vi "GLIMPSE Sequence Player.vi"() -> (8 "Sequence Range":cluster{i32, i32})   [LabVIEW 2016]
doc: "Allows the user to view and analyze a sequence of video stored as a temporary file on the disk. Also includes tools for setting areas of interest, manual tracking, automatic tracking by image fitting, etc."
uses:
  Header file data.ctl
  Seq file v 1/Offset table.ctl
  Seq file v 1/Offset.ctl
  Seq file v 1/file number.ctl
  Header2 file data.ctl
  <vilib>/vision/Image Controls.llb/IMAQ Image.ctl
  GLIMPSE Globals.vi
  <vilib>/Utility/file.llb/Write To Spreadsheet File (I64).vi
  AOI/AOI List Globals.vi
  <vilib>/Utility/NIReport.llb/NI_ReportGenerationCore.lvlib
panel:
  out "Header2 data":T1
  in  "Exit":bool
  out "Acquisition refnum array":refnum<file>[](array[refnum])
  out "file path":path
  out "Header data":T2 {"Pixel depth" items=["8 bits", "16 bits", "Float", "Complex", "RGB", "HSL"]; "time of 1st frame, \nsec since 1/1/04" format="%.2f"}
  in  "Change File":bool
  in  "Tab Control":T6(tab)
  in  "Overlay?":bool=TRUE caption="Loop?"
  in  "Frames to Step":u32=1 min=1 step=1
  in  "# Display\nWindows":i32=1 min=0 max=8 step=1
  in  "Delay between frames (msec)":i32=33 min=0 max=2147483600 step=100
  in  "Stop!":bool
  out "Time after 1st\nFrame (ms)":u32
  out "Mode":T7(ring)
  out "Time\nStamp":u32
  in  "Step Backward":bool
  in  "Step Forward":bool
  in  "Play Backward":bool
  in  "Play Forward":bool
  in  "Go to End":bool
  in  "Go to Begin":bool
  in  "Toggle beg/end":bool
  in  "Set end":bool
  in  "Set begin":bool
  in  "Loop?":bool=TRUE
  in  "Range Enabled":bool=TRUE caption="Restrict playback to range"
  in  "Frame Number":cluster{u32, u32}(slide)={10, 1} scale=1.0..3558.0
  in  "Current Frame Number":u32(slide) max=3558 scale=1.0..3558.0
  out "Rev bkd":bool
  out "Fwd bkd":bool
  out "Stop bkgd":bool
  out "Filter":u16
  out "Field":u16
  out "Lasers":bool[](array[boolean])
  out "Flow":dbl
  out "Temp":dbl
  in  "Total FOVs":i16=4
  in  "Display FOV number":i16(slide)=1 min=1 scale=1.0..4.0
  in  "FOV Mode":T8(ring)=enum."Display all frames"
  in  "Printer":u16(ring) items=["zippy", "Send To OneNote 2010", "prism", "Microsoft XPS Document Writer", "Fax"]
  in  "Track by Curve Fitting to AOIs":bool
  in  "Print Image":bool
  in  "Save Portion of Current Frame":bool
  in  "Save Sequence":bool
  in  "Set/Modify AOIs (F8)":bool
  in  "Clear All":bool
  in  "Erase Last Row":bool
  out "Tracking Output File":path
  out "Number of Points":i16
  in  "Table":string[][](table)
  out "Pixel depth":u32(ring) items=["8 bits", "16 bits", "Float", "Complex", "RGB", "HSL"]
  out "Number of Frames":u32
  out "Frame width":i32
  out "Frame height":i32
  out "Camera":string
  out "Microscope":string
  out "Microscope software version":string
  out "Filter names":string[](array[string])
  out "Laser names":string[](array[string])
  # "These parameters are not for interactive use:"
  # "1"
  # "1"
  # "(F1)"
  # "(F2)"
  # "(F3)"
  # "(F4)"
  # "(F12)"
  # "Begin"
  # "Set"
  # "End"
  # "To add an (X, Y, T) point to table, click on image #1 with the point tool (\"+\")."
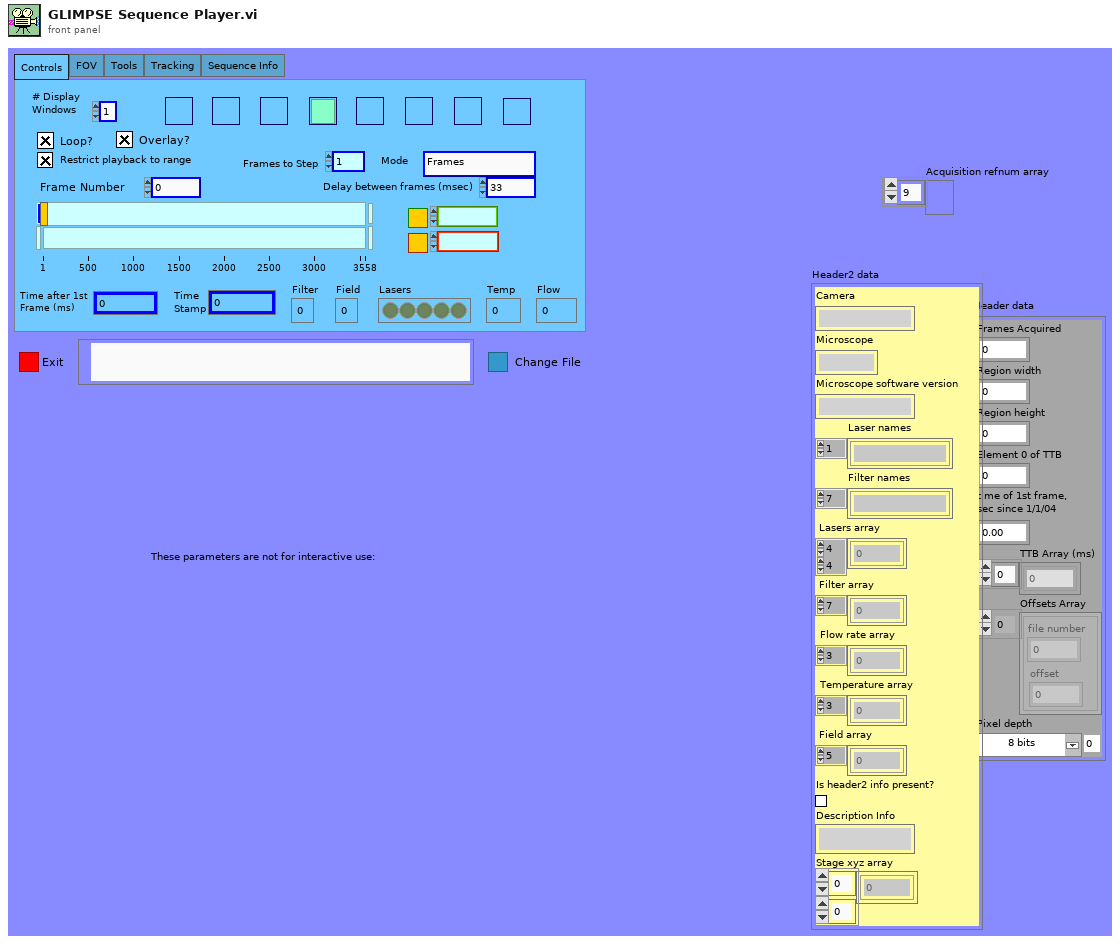
[diagram p1: front panel]
types:
  T1 = typedef "Header2 file data.ctl" = cluster{"Camera":string, "Microscope":string, "Microscope software version":string, "Laser names":string[], "Filter names":string[], "Lasers array":u16[][], "Filter array":u16[], "Flow rate array":dbl[], "Temperature array":dbl[], "Field array":u16[], "Is header2 info present?":bool, "Description Info":string, "Stage xyz array":dbl[][]}
  T2 = typedef "Header file data.ctl" = cluster{"Frames Acquired":u32, "Region width":i32, "Region height":i32, "Element 0 of TTB":u32, "time of 1st frame, \nsec since 1/1/04":dbl, "TTB Array (ms)":u32[], "Offsets Array":T3, "Pixel depth":u32}
  T3 = typedef "Offset table.ctl" = cluster{"offset":T4, "file number":T5}[]
  T4 = typedef "Offset.ctl" = i32
  T5 = typedef "file number.ctl" = u8
  T6 = enum32{"Controls", "FOV", "Tools", "Tracking", "Sequence Info"}
  T7 = enum16{"Frames", "Fields, Odd 1st", "Fields, Even 1st", "Fields, Averaged"}
  T8 = enum16{"Display one field of view", "Display all frames"}
  T9 = typedef "IMAQ Image.ctl" = refnum<image>
  T10 = enum32{"No Selection", "Point", "Line", "Rectangle", "Oval", "Polygon", "Free", "Unused1", "Zoom", "Unused2", "Broken Line", "Free Hand Line"}
  T11 = enum32{"No  event", "Click event", "Draw event", "Move event", "Size event", "Scroll event", "Activate event", "Close event", "Reserved"}[]
  T12 = cluster{"# of Frames Out (Log)":u32, "Current Frame Number":u32}
  T13 = cluster{"Left":i32, "Top":i32, "Right":i32, "Bottom":i32}
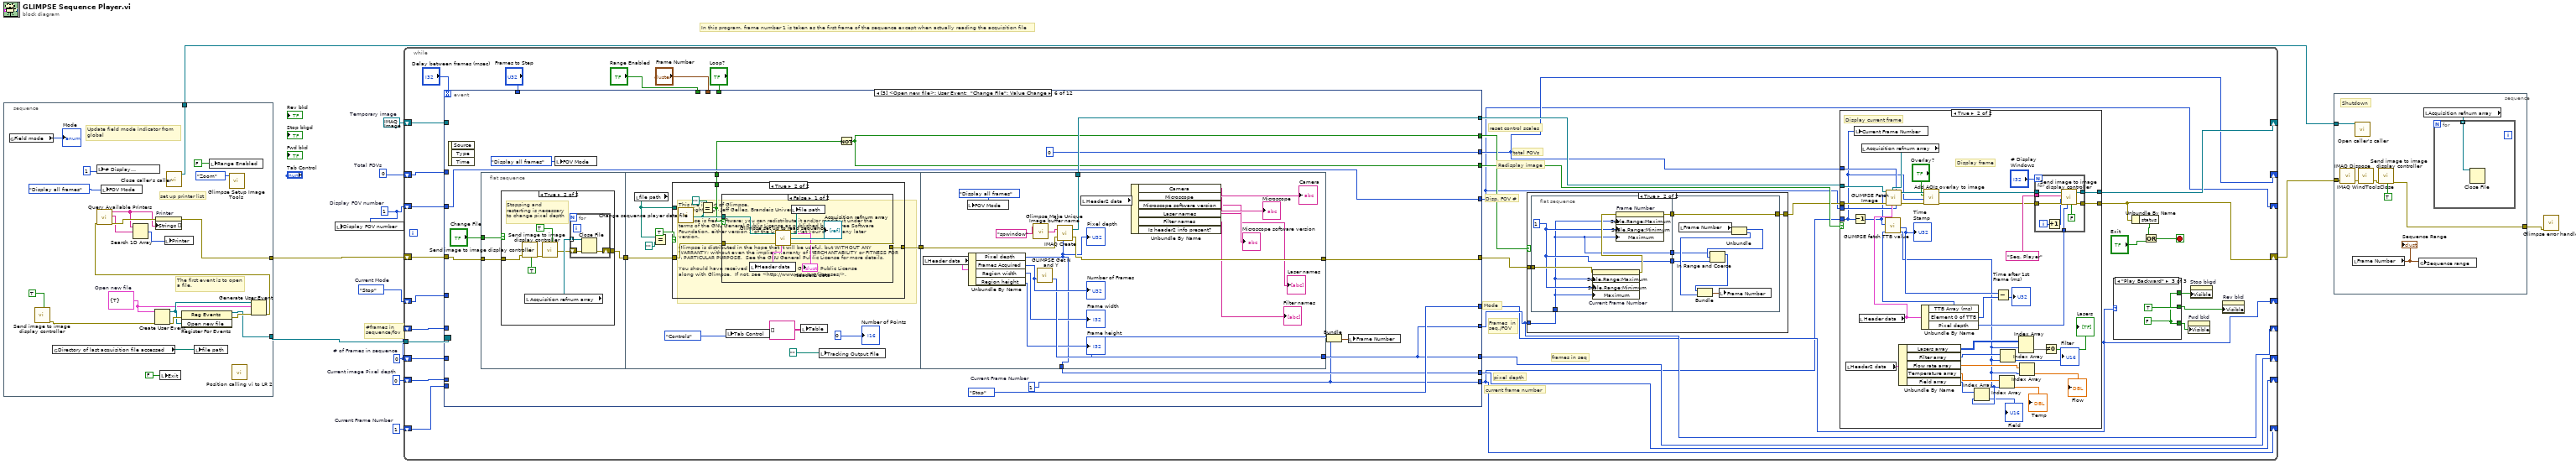
[diagram p0: block diagram]
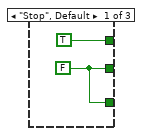
[diagram p2: hidden frame]
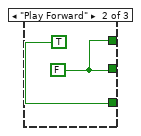
[diagram p3: hidden frame]
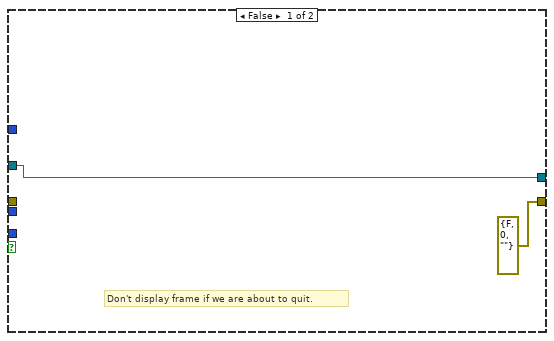
[diagram p4: hidden frame]
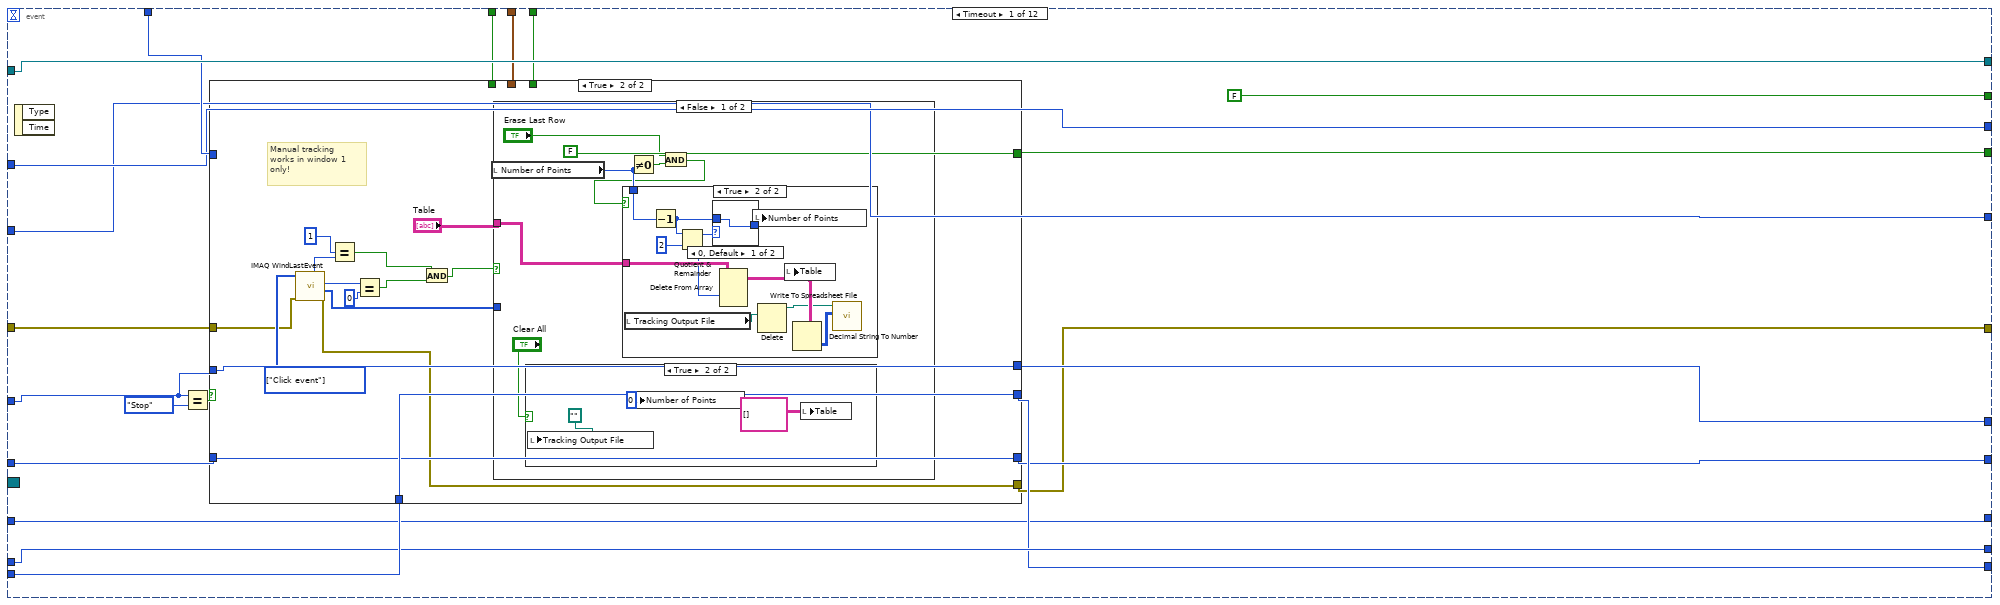
[diagram p6: hidden frame]
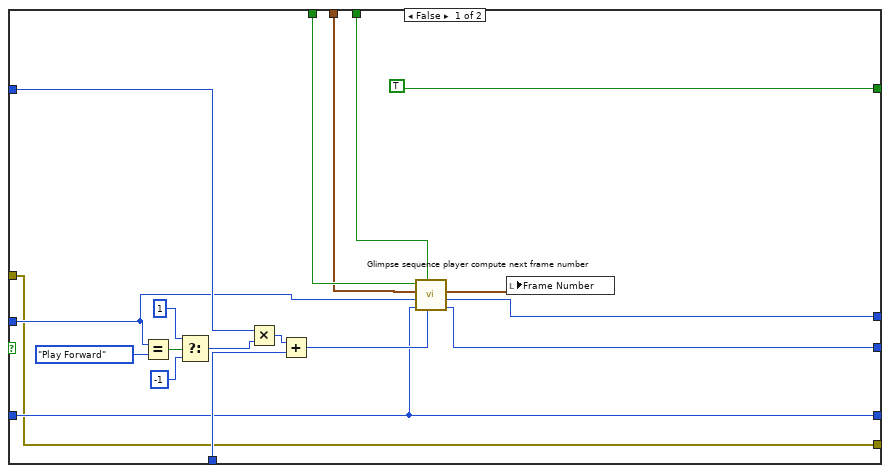
[diagram p7: hidden frame]
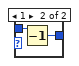
[diagram p10: hidden frame]
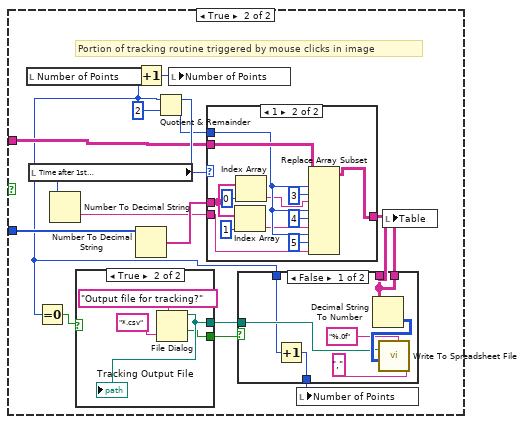
[diagram p11: hidden frame]
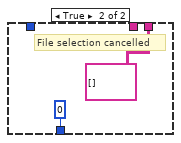
[diagram p12: hidden frame]
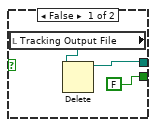
[diagram p13: hidden frame]
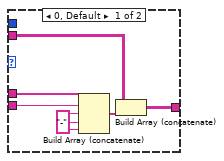
[diagram p14: hidden frame]
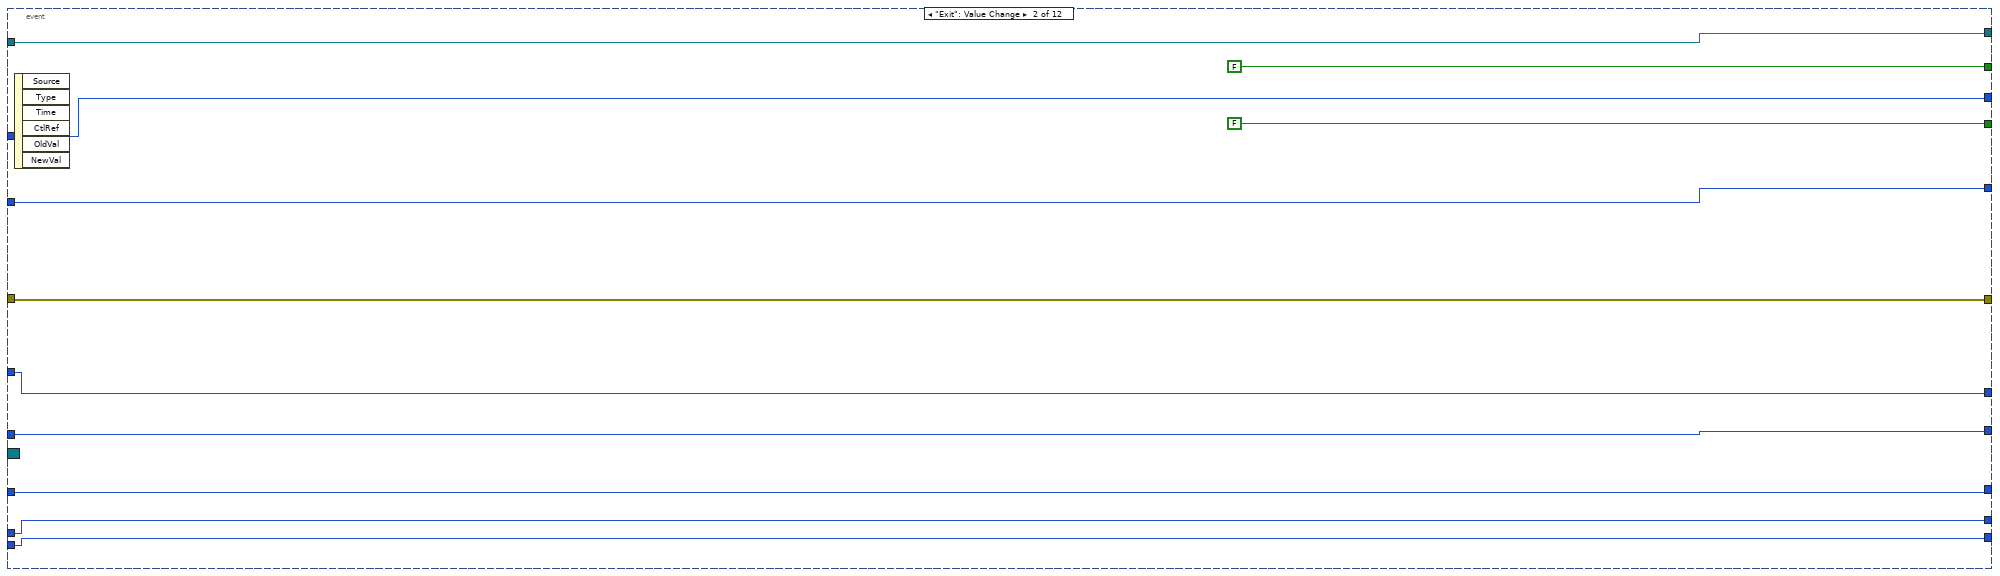
[diagram p15: hidden frame]
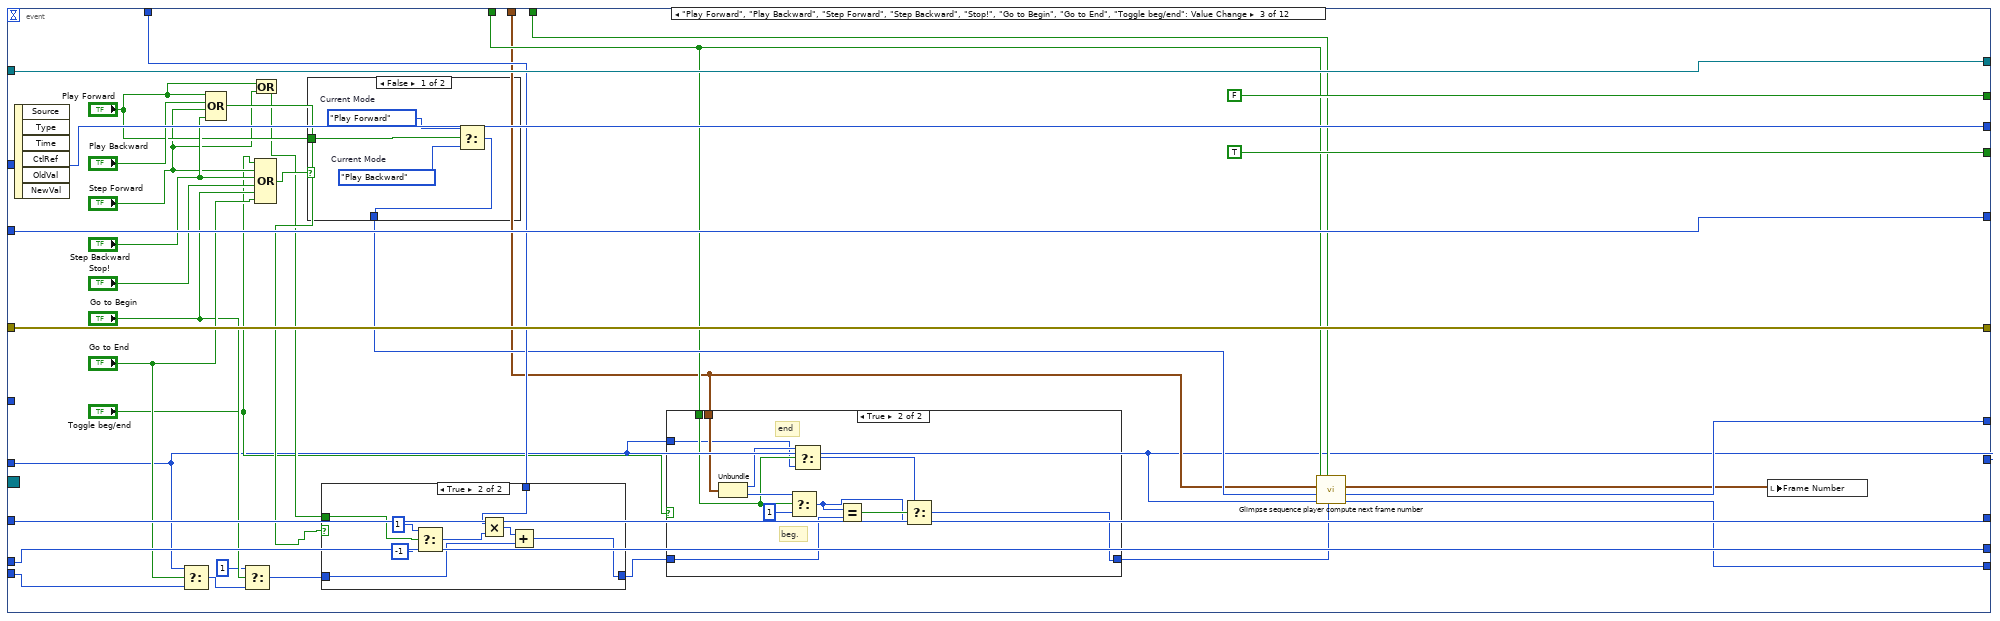
[diagram p16: hidden frame]
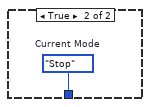
[diagram p19: hidden frame]
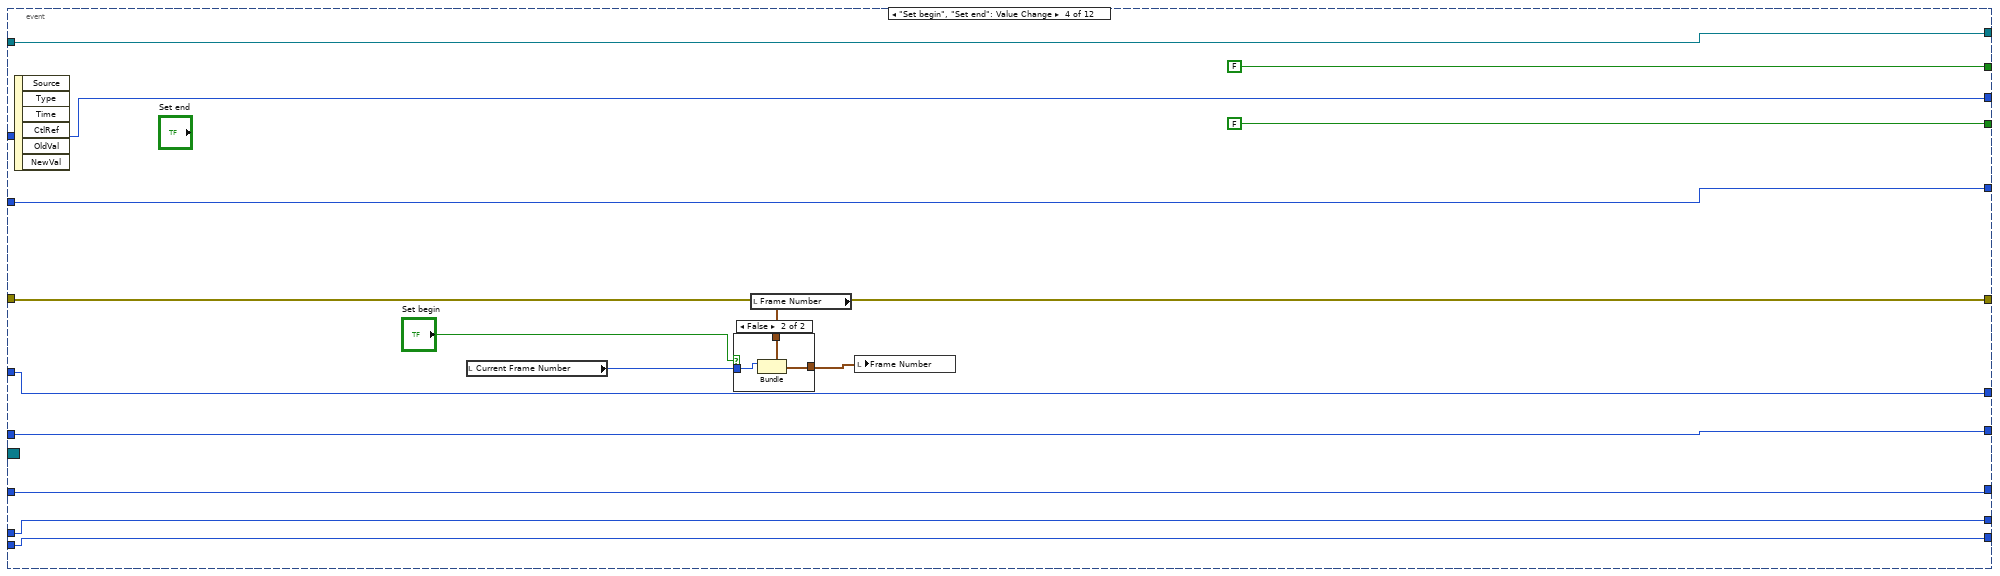
[diagram p20: hidden frame]
diagram:
  w3 = u32 0  # # of Frames in sequence
  w6 = T9 refnum  # Temporary image
  w4 = i16 1  # Display FOV number
  w7 = i16 0  # Total FOVs
  w8 = u32 0  # Current image Pixel depth
  w11 = u32 1  # Current Frame Number
  w5 = enum16{"Stop", "Play Forward", "Play Backward"}."Stop"  # Current Mode
  # "This file is part of Glimpse. \nCopyright 2014 Jeff Gelles, Brandeis University.    \n\nGlimpse is free software: you can redistribute it and/or modify it under the \nterms of the GNU General Public License as published by the Free Software \nFoundation, either version 3 of the License, or (at your option) any later \nversion.\n\nGlimpse is distributed in the hope that it will be useful, but WITHOUT ANY \nWARRANTY; without even the implied warranty of MERCHANTABILITY or FITNESS FOR \nA PARTICULAR PURPOSE.  See the GNU General Public License for more details.\n\nYou should have received a copy of the GNU General Public License\nalong with Glimpse.  If not, see <http://www.gnu.org/licenses/>."
  # "#frames in\nsequence/fov"
  # "In this program, frame number 1 is taken as the first frame of the sequence except when actually reading the acquisition file"
  n1 = stacked-sequence {
    tunnel: [w32] -> w12
    tunnel: [w21] -> w10
    tunnel: [w17] -> w9
    frame #0 {
      w14 = cluster{"dummy":bool} {"dummy"=TRUE}  # Open new file
      # "Update field mode indicator from\nglobal"
      # "The first event is to open\na file."
      # "set up printer list"
      n2 = global read "GLIMPSE Globals.vi" "Field mode"() -> (→"Mode":T7)
      n3 = call "Send image to image display controller.vi"("Start display controller?"=TRUE ("Quit display controller?")) -> ("error out"=w18:errorcluster)  [unwired: 6 in, 3 out]
      n4 = global read "GLIMPSE Globals.vi" "Directory of last acquisition file accessed"() -> (w25:path)
      n5 = local write "# Display\nWindows"(1 ("# Display\nWindows")) -> ()
      n6 = local write "FOV Mode"(T8."Display all frames" ("FOV Mode")) -> ()
      n7 = Create User Event(user event datatype=w14, error in=w18) -> (user event=w22:refnum<user-event>, error out=w24:errorcluster)
      n8 = local write "Exit"(FALSE ("Exit")) -> ()
      n9 = call "Close caller's caller.vi"() -> ("vi reference"=w32:refnum<vi>)  [unwired: 1 in, 7 out]
      n10 = register-events(error in=w24, w22) -> (reference out=w21:refnum<event-registration>, error out=w23:errorcluster)  [unwired: 1 in]
      n11 = local write "file path"(w25) -> ()
      n12 = local write "Range Enabled"(FALSE ("Exit")) -> ()
      n13 = call "Glimpse Setup Image Tools"("Default Tool"=T10."Zoom") -> ()  [unwired: 1 in, 3 out]
      n14 = call "Position calling vi to LR 2.vi"() -> ()  [unwired: 2 in, 4 out]
      n15 = Generate User Event(user event=w22, event data cluster=w14, error in=w23) -> (error out=w20:errorcluster)  [unwired: 1 in, 1 out]
      n16 = call <vilib>:"Query Available Printers.vi"("error in (no error)"=w20) -> ("error out"=w30:errorcluster, "default printer"=w29:string, "system configured printers"=w28:string[])  [unwired: 8 out]
      n17 = Search 1D Array(1D array=w28, element=w29) -> (index of element=w27:i32)  [unwired: 1 out]
      n18 = property on="Printer" class="Ring (strict)"(error in=w30, "Strings []"=w28) -> (error out=w17:errorcluster)  [unwired: 1 in, 1 out]
      n19 = local write "Printer"(w27) -> ()
    }
  }
  n20 = local write "Display FOV number"(w4) -> ()
  n21 = while {
    shift-right: [w34] -> _
    shift-left: w11 -> [w66]
    tunnel: w10 -> [w68]
    shift-right: [w43] -> w2
    shift-left: w9 -> [w67]
    shift-right: [w56] -> _
    shift-left: w6 -> [w61]
    shift-right: [w65] -> _
    shift-left: w8 -> [w64]
    shift-right: [w47] -> _
    shift-left: w7 -> [w63]
    shift-right: [w46] -> _
    shift-left: w4 -> [w62]
    shift-right: [w38] -> _
    shift-left: w5 -> [w60]
    shift-right: [w55] -> _
    shift-left: w3 -> [w59]
    shift-right: [w39] -> _
    shift-left: w3 -> [w45]
    stop <- w44 stop-if-true
    (unwired) cluster{string, u32}[] [] ("Images")
    # "pixel depth"
    # "frames in seq"
    # "Frames  in\nseq./FOV"
    # "Mode"
    # "Disp. FOV #"
    # "total FOVs"
    # "current frame number"
    # "Redisplay image"
    # "reset control scales"
    n22 = event shown="[5] <Open new file>: User Event;  \"Change File\": Value Change" {
      selector: w68 -> [_ _ _ _ _ _ _ _ _ _ _ _]
      dyn-events: _ -> [_ _ _ _ _ _ _ _ _ _ _ _]
      timeout: "Delay between frames (msec)" -> [_ _ _ _ _ _ _ _ _ _ _ _]
      tunnel: w67 -> [w142 w273 w310 w348 w367 w399 w505 w528 w552 w581 w595 w623]
      tunnel: [w159 w280 w314 w355 w373 w396 w467 w530 w551 w585 w596 w624] -> w57
      tunnel: [w141 w273 w310 w348 w367 w395 w474 w528 w539 w581 w594 w623] -> w49
      tunnel: [FALSE ("Reset control scales?") FALSE ("Reset control scales?") FALSE ("Reset control scales?") FALSE ("Reset control scales?") FALSE ("Reset control scales?") w384 w472 w532 w554 w587 TRUE ("Reset control scales?") w628] -> w58
      tunnel: w66 -> [w154 w279 w303 w354 w372 _ w464 w534 w549 w584 w602 _]
      tunnel: [w151 w279 w291 w354 w372 w387 w464 w534 w549 w584 w599 "Current Frame Number"] -> w34
      tunnel: [w152 w278 w313 w353 w371 w392 w475 w533 w548 w583 w600 w626] -> w65
      tunnel: w64 -> [w152 w278 w313 w353 w371 _ w475 w533 w548 w583 w600 w626]
      tunnel: w63 -> [w153 w270 w307 w345 w364 _ w470 w529 w544 w580 _ w619]
      tunnel: w62 -> [w144 w274 w311 w349 w368 w390 w469 w527 w541 w578 _ w620]
      tunnel: w61 -> [w159 w280 w314 w355 w373 _ w468 w530 w551 w585 w596 w624]
      tunnel: w60 -> [w156 w275 _ w350 _ _ _ _ w550 w579 w593 w622]
      tunnel: [w146 w275 w289 w350 w362 enum16{"Stop", "Play Forward", "Play Backward"}."Stop" ("Current Mode") enum16{"Stop", "Play Forward", "Play Backward"}."Stop" ("Current Mode") enum16{"Stop", "Play Forward", "Play Backward"}."Stop" ("Current Mode") w550 w579 w593 w622] -> w38
      tunnel: [w145 w277 w312 w352 w370 w388 w465 w525 w547 w582 w598 w625] -> w55
      tunnel: w59 -> [w145 w277 w312 w352 w370 _ w465 w525 w547 w582 w598 w625]
      tunnel: [w153 w270 w307 w345 w364 i16 0 ("Total FOVs") w470 w529 w544 w580 w606 w619] -> w47
      tunnel: [w144 w274 w311 w349 w368 w390 w469 w527 w541 w578 w605 w620] -> w46
      tunnel: [w143 w276 w281 w351 w369 w388 w466 w526 w546 w577 w603 w621] -> w39
      tunnel: [w157 FALSE ("Redisplay image") TRUE ("Redisplay image") FALSE ("Redisplay image") FALSE ("Redisplay image") w384 w471 w531 w553 w586 TRUE ("Redisplay image") w627] -> w50
      tunnel: w45 -> [w150 w276 w281 w351 w369 _ w466 w526 w546 w577 _ w621]
      tunnel: "Frames to Step" -> [w155 _ w295 _ _ _ _ _ _ _ _ _]
      tunnel: "Loop?" -> [w149 _ w288 _ _ _ _ _ _ _ _ _]
      tunnel: "Range Enabled" -> [w148 _ w283 _ _ _ _ _ _ _ _ _]
      tunnel: "Frame Number" -> [w147 _ w282 _ w363 _ _ _ _ _ _ _]
      event Timeout {
        n23 = event-data() -> ()  [unwired: 3 out]
        n24 = Equal?(x=w156, y=enum16{"Stop", "Play Forward", "Play Backward"}."Stop") -> (x = y?=w161:bool)
        n25 = case shown="True" w161 {
          tunnel: [TRUE ("Reset control scales?") FALSE ("Reset control scales?")] -> w157
          tunnel: w156 -> [w167 w194]
          tunnel: w155 -> [w177 _]
          tunnel: w154 -> [w172 w195]
          tunnel: [w165 w195] -> w151
          tunnel: w150 -> [w163 w193]
          tunnel: w149 -> [w170 _]
          tunnel: w148 -> [w169 _]
          tunnel: w147 -> [w168 _]
          tunnel: [w164 w194] -> w146
          tunnel: [w163 w193] -> w143
          tunnel: w142 -> [w162 w182]
          tunnel: [w162 w181] -> w141
          frame False {
            n26 = Equal?(x=w167, y=enum16{"Stop", "Play Forward", "Play Backward"}."Play Forward") -> (x = y?=w178:bool)
            n27 = Select(t=1, s=w178, f=-1) -> (s? t:f=w176:i32)
            n28 = Multiply(x=w177, y=w176) -> (x*y=w173:u32)
            n29 = Add(x=w173, y=w172) -> (x+y=w166:u32)
            n30 = call "Glimpse sequence player compute next frame number.vi"("Current Frame Number"=w166, "Loop?"=w170, "# of Frames in sequence/FOV"=w163, "Current Mode"=w167, "Range In"=w168, "Range Enabled"=w169) -> ("Current Frame Number Out"=w165:u32, "Current Mode Out"=w164:enum16{"Stop", "Play Forward", "Play Backward"}, "Range Out"=w171:cluster{"Max":u32, "Min":u32})  [unwired: 1 out]
            n31 = local write "Frame Number"(w171) -> ()
          }
          frame True {
            w191 = T11 [enum."Click event"] items=["No  event", "Click event", "Draw event", "Move event", "Size event", "Scroll event", "Activate event", "Close event", "Reserved"] ("Events list (all)")
            # "Manual tracking \nworks in window 1\nonly!"
            n32 = call "IMAQ WindLastEvent"("error in (no error)"=w182, "Events list (all)"=w191) -> ("error out"=w181:errorcluster, "Coordinates"=w185:i32[], "Tool"=w190:i32, "Window Number (0...15)"=w192:i32)  [unwired: 6 out]
            n33 = Equal?(x=1 ("Window Number (0...15)"), y=w192) -> (x = y?=w187:bool)
            n34 = Equal?(x=w190, y=0) -> (x = y?=w188:bool)
            n35 = And(x=w187, y=w188) -> (x .and. y?=w186:bool)
            n36 = case shown="False" w186 {
              tunnel: w185 -> [_ w231]
              tunnel: "Table" -> [w201 w225]
              frame False {
                n37 = local read "Number of Points"() -> (w200:i16)
                n38 = case shown="True" "Clear All" {
                  frame False {
                  }
                  frame True {
                    n39 = local write "Tracking Output File"(path "") -> ()
                    n40 = local write "Number of Points"(i16 0 ("Number of Points")) -> ()
                    n41 = local write "Table"(string[][] []) -> ()
                  }
                }
                n42 = Not Equal To 0?(x=w200) -> (x != 0?=w199:bool)
                n43 = And(x="Erase Last Row", y=w199) -> (x .and. y?=w198:bool)
                n44 = case shown="True" w198 {
                  tunnel: w201 -> [_ w212]
                  tunnel: w200 -> [_ w207]
                  frame False {
                  }
                  frame True {
                    n45 = local read "Tracking Output File"() -> (w206:path)
                    n46 = Decrement(x=w207) -> (x-1=w215:i16)
                    n47 = Quotient & Remainder(x=w215, y=i16 2) -> (x-y*floor(x/y)=w213:i16, floor(x/y)=w211:i16)
                    n48 = case shown="0, Default" w213 {
                      tunnel: w215 -> [w217 w219]
                      tunnel: [w217 w218] -> w214
                      frame 0, Default {
                      }
                      frame 1 {
                        n49 = Decrement(x=w219) -> (x-1=w218:i16)
                      }
                    }
                    n50 = Delete From Array(array=w212, index (row)=w211) -> (array with subset deleted=w210:string[][])  [unwired: 2 in, 1 out]
                    n51 = local write "Number of Points"(w214) -> ()
                    n52 = Delete(path (use dialog)=w206) -> (deleted path=w209:path)  [unwired: 1 in, 5 out]
                    n53 = local write "Table"(w210) -> ()
                    n54 = Decimal String To Number(string=w210) -> (number=w208:i32[][])  [unwired: 3 out]
                    n55 = call-poly <vilib>:"Write To Spreadsheet File.vi"("2D data"=w208, "file path (dialog if empty)"=w209) -> ()  [unwired: 4 in, 3 out]
                  }
                }
              }
              frame True {
                # "Portion of tracking routine triggered by mouse clicks in image"
                n56 = local read "Number of Points"() -> (w222:i16)
                n57 = local read "Time after 1st\nFrame (ms)"() -> (w232:u32)
                n58 = Equal To 0?(x=w222) -> (x = 0?=w227:bool)
                n59 = Number To Decimal String(number=w232) -> (decimal integer string=w229:string)  [unwired: 1 out]
                n60 = case shown="True" w227 {
                  tunnel: [w246 w249] -> w223
                  tunnel: [FALSE ("cancelled") w248] -> w224
                  frame False {
                    n61 = local read "Tracking Output File"() -> (w247:path)
                    n62 = Delete(path (use dialog)=w247) -> (deleted path=w246:path)  [unwired: 1 in, 5 out]
                  }
                  frame True {
                    n63 = File Dialog(6:"*.csv" ("pattern"), 7:"Output file for tracking?" ("prompt")) -> (1:w248:bool, 3:w249:path)  [unwired: 1 in, 6 out]
                    "Tracking Output File" <- w249
                  }
                }
                n64 = Increment(x=w222) -> (x+1=w234:i16)
                n65 = Number To Decimal String(number=w231) -> (decimal integer string=w230:string[])  [unwired: 1 in]
                n66 = Quotient & Remainder(x=w222, y=i16 2) -> (x-y*floor(x/y)=w233:i16, floor(x/y)=w228:i16)
                n67 = local write "Number of Points"(w234) -> ()
                n68 = case shown="1" w233 {
                  tunnel: w225 -> [w257 w269]
                  tunnel: [w254 w268] -> w226
                  tunnel: w230 -> [w253 w262]
                  tunnel: w229 -> [w252 w263]
                  tunnel: w228 -> [_ w264]
                  frame 0, Default {
                    w255 = "-"
                    n69 = Build Array (concatenate)(w253, w252, w255, w255, w255) -> (w256:string[])
                    n70 = Build Array (concatenate)(w257, w256) -> (w254:string[][])
                  }
                  frame 1 {
                    n71 = Index Array(array=w262, index=1 ("Index")) -> (element=w258:string)
                    n72 = Index Array(array=w262, index=0 ("Index")) -> (element=w259:string)
                    n73 = Replace Array Subset(array=w269, new element #1=w259, index (row) #1=w264, index (col) #1=3 ("Disabled Index (col)"), new element #2=w258, index (row) #2=w264, index (col) #2=4 ("Index (col)"), new element #3=w263, index (row) #3=w264, index (col) #3=5 ("Index (col)")) -> (w268:string[][])
                  }
                }
                n74 = case shown="False" w224 {
                  tunnel: w226 -> [w238 _]
                  tunnel: w223 -> [w241 _]
                  tunnel: w222 -> [w240 _]
                  tunnel: [w239 i16 0] -> w221
                  tunnel: [w238 string[][] []] -> w220
                  frame False {
                    n75 = Increment(x=w240) -> (x+1=w239:i16)
                    n76 = Decimal String To Number(string=w238) -> (number=w242:i32[][])  [unwired: 3 out]
                    n77 = call-poly <vilib>:"Write To Spreadsheet File.vi"("delimiter (\\t)"="," ("delimiter (Tab)"), "format (%d)"="%.0f" ("format (%.3f)"), "2D data"=w242, "file path (dialog if empty)"=w241) -> ()  [unwired: 3 in, 2 out]
                  }
                  frame True {
                    # "File selection cancelled"
                  }
                }
                n78 = local write "Number of Points"(w221) -> ()
                n79 = local write "Table"(w220) -> ()
              }
            }
          }
        }
      }
      event "Exit": Value Change {
        n80 = event-data() -> ()  [unwired: 7 out]
      }
      event "Play Forward", "Play Backward", "Step Forward", "Step Backward", "Stop!", "Go to Begin", "Go to End", "Toggle beg/end": Value Change {
        n81 = event-data() -> ()  [unwired: 7 out]
        n82 = Select(t=w281, s="Go to End", f=w303) -> (s? t:f=w301:u32)
        n83 = Compound Arithmetic op=OR("Play Forward", "Play Backward", "Step Forward", "Step Backward") -> (w297:bool)
        n84 = Select(t=u32 1, s="Go to Begin", f=w301) -> (s? t:f=w296:u32)
        n85 = Or(x="Play Forward", y="Step Forward") -> (x .or. y?=w292:bool)
        n86 = Compound Arithmetic op=OR("Toggle beg/end", "Step Forward", "Step Backward", "Stop!", "Go to Begin", "Go to End") -> (w305:bool)
        n87 = case shown="False" w305 {
          tunnel: [w336 w340] -> w290
          tunnel: "Play Forward" -> [w339 _]
          frame False {
            w337 = enum16{"Stop", "Play Forward", "Play Backward"}."Play Backward"  # Current Mode
            w338 = enum16{"Stop", "Play Forward", "Play Backward"}."Play Forward"  # Current Mode
            n88 = Select(t=w338, s=w339, f=w337) -> (s? t:f=w336:enum16{"Stop", "Play Forward", "Play Backward"})
          }
          frame True {
            w340 = enum16{"Stop", "Play Forward", "Play Backward"}."Stop"  # Current Mode
          }
        }
        n89 = case shown="True" w297 {
          tunnel: w296 -> [w327 w330]
          tunnel: [w327 w329] -> w285
          tunnel: w295 -> [_ w331]
          tunnel: w292 -> [_ w328]
          frame False {
          }
          frame True {
            n90 = Select(t=1, s=w328, f=-1) -> (s? t:f=w333:i32)
            n91 = Multiply(x=w331, y=w333) -> (x*y=w335:u32)
            n92 = Add(x=w335, y=w330) -> (x+y=w329:u32)
          }
        }
        n93 = case shown="True" "Toggle beg/end" {
          tunnel: w285 -> [w315 w325]
          tunnel: [w315 w316] -> w284
          tunnel: w283 -> [_ w320]
          tunnel: w282 -> [_ w323]
          tunnel: w281 -> [_ w318]
          frame False {
          }
          frame True {
            # "end"
            # "beg."
            n94 = Unbundle(w323) -> (w319:u32, w322:u32)
            n95 = Select(t=w322, s=w320, f=u32 1) -> (s? t:f=w321:u32)
            n96 = Select(t=w319, s=w320, f=w318) -> (s? t:f=w317:u32)
            n97 = Equal?(x=w321, y=w325) -> (x = y?=w324:bool)
            n98 = Select(t=w317, s=w324, f=w321) -> (s? t:f=w316:u32)
          }
        }
        n99 = call "Glimpse sequence player compute next frame number.vi"("Current Frame Number"=w284, "Loop?"=w288, "# of Frames in sequence/FOV"=w281, "Current Mode"=w290, "Range In"=w282, "Range Enabled"=w283) -> ("Current Frame Number Out"=w291:u32, "Current Mode Out"=w289:enum16{"Stop", "Play Forward", "Play Backward"}, "Range Out"=w287:cluster{"Max":u32, "Min":u32})  [unwired: 1 out]
        n100 = local write "Frame Number"(w287) -> ()
      }
      event "Set begin", "Set end": Value Change {
        n101 = event-data() -> ()  [unwired: 7 out]
        n102 = local read "Current Frame Number"() -> (w343:u32)
        n103 = local read "Frame Number"() -> (w342:cluster{u32, u32})
        n104 = case shown="False" "Set begin" {
          tunnel: [w358 w361] -> w344
          tunnel: w343 -> [w357 w359]
          tunnel: w342 -> [w356 w360]
          frame True {
            n105 = Bundle(cluster=w356, w357) -> (w358:cluster{u32, u32})  [unwired: 1 out]
          }
          frame False {
            n106 = Bundle(cluster=w360, w359) -> (w361:cluster{u32, u32})  [unwired: 1 out]
          }
        }
        n107 = local write "Frame Number"(w344) -> ()
      }
      event "Track by Curve Fitting to AOIs": Value Change {
        n108 = event-data() -> ()  [unwired: 7 out]
        n109 = flat-sequence {
          tunnel: [enum16{"Stop", "Play Forward", "Play Backward"}."Stop" ("Current Mode")] -> w362
          tunnel: w363 -> [w374]
          frame #0 {
            n110 = global read "GLIMPSE Globals.vi" "Current window Black/White Levels"() -> (w375:cluster{ext, ext})
            n111 = local read "Acquisition refnum array"() -> (w381:refnum<file>[])
            n112 = local read "Header data"() -> (w376:T2)
            n113 = Unbundle(w374) -> (w380:u32, w379:u32)
            n114 = Unbundle(w375) -> (w378:ext, w377:ext)
            n115 = call "fit aois.vi"("End frame"=w380, "White level"=w377, "Header Info"=w376, "Start frame"=w379, "Black level"=w378, "Acquisition refnum array"=w381) -> ()  [unwired: 5 out]
          }
          frame #1 {
            n116 = call "IMAQ WindToolsShow"() -> ("error out"=w383:errorcluster)  [unwired: 3 in, 3 out]
            n117 = call <vilib>:"Simple Error Handler.vi"("error in (no error)"=w383) -> ()  [unwired: 1 in, 8 out]
          }
        }
      }
      event User Event; "Change File": Value Change {
        w387 = u32 1  # Current Frame Number
        n118 = event-data() -> ()  [unwired: 4 out]
        n119 = flat-sequence {
          tunnel: w399 -> [w402]
          tunnel: [w401] -> w398
          tunnel: "Change File" -> [w400]
          tunnel: w398 -> [w421]
          tunnel: [w416] -> w397
          tunnel: [w414] -> w385
          tunnel: w397 -> [w460]
          tunnel: [w459] -> w396
          tunnel: [w458] -> w395
          tunnel: [w452] -> w392
          tunnel: [w456] -> w388
          frame #0 {
            n120 = case shown="True" w400 {
              tunnel: w402 -> [w403 w408]
              tunnel: [w403 w407] -> w401
              frame False {
              }
              frame True {
                # "Stopping and \nrestarting is necessary\nto change pixel depth"
                n121 = call "Send image to image display controller.vi"("error in"=w408, "Quit display controller?"=TRUE) -> ("error out"=w404:errorcluster)  [unwired: 5 in, 3 out]
                n122 = local read "Acquisition refnum array"() -> (w410:refnum<file>[])
                n123 = call "Send image to image display controller.vi"("error in"=w404, "Start display controller?"=TRUE ("Quit display controller?")) -> ("error out"=w409:errorcluster)  [unwired: 5 in, 3 out]
                n124 = for {
                  tunnel: w410 -> [w413] mode=indexing
                  shift-right: [w411] -> w407
                  shift-left: w409 -> [w412]
                  n125 = Close File(refnum=w413, error in=w412) -> (error out=w411:errorcluster)  [unwired: 1 out]
                }
              }
            }
          }
          frame #1 {
            n126 = local read "file path"() -> (w423:path)
            n127 = Equal?(x=w423, y=path "") -> ()  [unwired: 1 out]
            n128 = case shown="True" TRUE {
              tunnel: w423 -> [w431 _]
              tunnel: w421 -> [w427 w434]
              tunnel: [w426 w433] -> w416
              tunnel: [FALSE w432] -> w414
              frame False {
                # "automatically open last file accessed"
                n129 = call "Glimpse set up to read sequence.vi"("acquisition directory path"=w431, "error in"=w427) -> ("Header2 file data out"=w424:T1, "Header file data out"=→"Header data":T2, "acquisition directory path out"=→"file path":path, "Acquisition refnum array"=w429:refnum<file>[], "error out"=w426:errorcluster)  [unwired: 1 out]
                n130 = local write "Acquisition refnum array"(w429) -> ()
                n131 = local write "Header2 data"(w424) -> ()
              }
              frame True {
                n132 = call "Change sequence player data file.vi"() -> ("File path out"=w436:path)  [unwired: 1 in, 4 out]
                n133 = Equal?(x=path "", y=w436) -> (x = y?=w432:bool)
                n134 = case shown="False" w432 {
                  tunnel: w436 -> [w443 _]
                  tunnel: w434 -> [w439 w445]
                  tunnel: [w438 w445] -> w433
                  frame False {
                    n135 = call "Glimpse set up to read sequence.vi"("acquisition directory path"=w443, "error in"=w439) -> ("Header2 file data out"=→"Header2 data":T1, "Header file data out"=w440:T2, "acquisition directory path out"=w442:path, "Acquisition refnum array"=→"Acquisition refnum array":refnum<file>[], "error out"=w438:errorcluster)  [unwired: 1 out]
                    n136 = local write "Header data"(w440) -> ()
                    n137 = local write "file path"(w442) -> ()
                  }
                  frame True {
                    n138 = local write "Exit"(TRUE ("Exit")) -> ()
                  }
                }
              }
            }
            n139 = local write "Tab Control"(enum32{"Controls", "FOV", "Tools", "Tracking"}."Controls" ("Tab Control")) -> ()
            n140 = local write "Table"(string[][] []) -> ()
            n141 = local write "Tracking Output File"(path "") -> ()
            "Number of Points" <- i16 0 ("Number of Points")
          }
          frame #2 {
            n142 = local read "Header data"() -> (w463:T2)
            n143 = local write "FOV Mode"(T8."Display all frames" ("FOV Mode")) -> ()
            n144 = Unbundle By Name(w463) -> ("Pixel depth"=w452:u32, "Frames Acquired"=w457:u32, "Region width"=→"Frame width":i32, "Region height"=→"Frame height":i32)
            "Number of Frames" <- w457
            "Pixel depth" <- w452
            n145 = call "Glimpse Make Unique Image buffer name.vi"("Buffer  base name"="spwindow" ("Image Name")) -> ("Image Name"=w462:string)  [unwired: 1 out]
            n146 = call "GLIMPSE Get N and Y.vi"("# of Frames In (Phys)"=w457) -> ("# of Frames Out (Log)"=w456:u32)  [unwired: 2 in, 4 out]
            n147 = call "IMAQ Create"("Image Name"=w462, "Image Type"=w452, "error in (no error)"=w460) -> ("New Image"=w459:T9, "error out"=w458:errorcluster)  [unwired: 1 in, 1 out]
            n148 = local read "Header2 data"() -> (w451:T1)
            n149 = Unbundle By Name(w451) -> ("Camera"=→"Camera":string, "Microscope"=→"Microscope":string, "Microscope software version"=→"Microscope software version":string, "Laser names"=→"Laser names":string[], "Filter names"=→"Filter names":string[])  [unwired: 1 out]
          }
        }
        n150 = local write "FOV Mode"(T8."Display all frames" ("FOV Mode")) -> ()
        n151 = Not(x=w385) -> (.not. x?=w384:bool)
        n152 = Bundle("# of Frames Out (Log)"=w388, "Current Frame Number"=w387) -> (w389:T12)  [unwired: 1 out]
        n153 = local write "Frame Number"(w389) -> ()
      }
      event "Set/Modify AOIs (F8)": Value Change {
        w471 = TRUE  # Redisplay image
        w472 = FALSE  # Reset control scales?
        n154 = event-data() -> ()  [unwired: 7 out]
        n155 = call "IMAQ Create"("Image Name"="Field1", "Image Type"=w475, "error in (no error)"=w505) -> ("New Image"=w509:T9, "error out"=w502:errorcluster)  [unwired: 1 in, 1 out]
        n156 = call "IMAQ Create"("Image Name"="Field2", "Image Type"=w475, "error in (no error)"=w502) -> ("New Image"=w508:T9, "error out"=w481:errorcluster)  [unwired: 1 in, 1 out]
        n157 = local read "Header data"() -> (w482:T2)
        n158 = local read "Frame Number"() -> (w499:cluster{u32, u32})
        n159 = global read "GLIMPSE Globals.vi" "Current window Black/White Levels"() -> (w493:cluster{ext, ext})
        n160 = Unbundle(w499) -> (w501:u32, w500:u32)
        n161 = Decrement(x=w501) -> (x-1=w498:u32)
        n162 = Decrement(x=w500) -> (x-1=w497:u32)
        n163 = local read "Acquisition refnum array"() -> (w496:refnum<file>[])
        n164 = call "GLIMPSE Fetch Image.vi"("Display FOV number"=w469, "Total FOVs"=w470, "Header file data"=w482, "Acqisition files refnums"=w496, "error in"=w481, "Logical Frame Number\n(starting with zero)"=w498, "Image In"=w509) -> ("error out"=w480:errorcluster, "Image Out"=w507:T9)  [unwired: 3 out]
        n165 = call "GLIMPSE Fetch Image.vi"("Display FOV number"=w469, "Total FOVs"=w470, "Header file data"=w482, "Acqisition files refnums"=w496, "error in"=w480, "Logical Frame Number\n(starting with zero)"=w497, "Image In"=w508) -> ("error out"=w479:errorcluster, "Image Out"=w506:T9)  [unwired: 3 out]
        n166 = Unbundle(w493) -> (w495:ext, w494:ext)
        n167 = call "Multiple AOIs.vi"("White level"=w494, "Black level"=w495, "First (or only) image (red)"=w507, "error in"=w479, "Second image (green)"=w506, "Image Type"=w475) -> ("error out"=w478:errorcluster)  [unwired: 5 out]
        n168 = call "IMAQ WindToolsShow"("error in (no error)"=w478) -> ("error out"=w491:errorcluster)  [unwired: 2 in, 3 out]
        n169 = local write "Tab Control"(enum32{"Controls", "FOV", "Tools", "Tracking"}."Controls" ("Tab Control")) -> ()
        n170 = call "IMAQ Dispose"("Image"=w507, "error in (no error)"=w491) -> ("error out"=w492:errorcluster)  [unwired: 1 in, 3 out]
        n171 = call "IMAQ Dispose"("Image"=w506, "error in (no error)"=w492) -> ("error out"=w477:errorcluster)  [unwired: 1 in, 3 out]
        n172 = Open VI Reference(vi path=path "GLIMPSE Sequence Player.vi", error in (no error)=w477) -> (vi reference=w488:refnum<vi>, error out=w487:errorcluster)  [unwired: 4 out]
        n173 = property class="VI"(reference=w488, error in=w487, "Front Panel Window:Is Frontmost"=TRUE) -> (reference out=w484:refnum<vi>, error out=w485:errorcluster)
        n174 = Close Reference(reference=w484, error in (no error)=w485) -> (error out=w476:errorcluster)
        n175 = global read "AOI List Globals.vi" "AOI List"() -> (w483:u16[][])
        n176 = for {
          tunnel: w483 -> [w516] mode=indexing
          shift-right: [w519] -> w474
          shift-left: w476 -> [w521]
          shift-right: [w523] -> w467
          shift-left: w468 -> [w524]
          i -> [w522]
          w514 = u32 16711680 ("Color")
          n177 = call "AOI to optional rectangle.vi"("x1, y1, x2, y2 with origin (0, 0)"=w516) -> ("Rectangle Out"=w513:T13)  [unwired: 4 out]
          n178 = Unbundle By Name(w513) -> ("Left"=w511:i32, "Top"=w510:i32)
          n179 = Increment(x=w522) -> (x+1=w517:i32)
          n180 = call "IMAQ Overlay Rectangle"("Color"=w514, "error in (no error)"=w521, "Rectangle"=w513, "Image"=w524) -> ("error out"=w520:errorcluster, "Image Out"=w518:T9)  [unwired: 2 in, 4 out]
          n181 = Number To Decimal String(number=w517) -> (decimal integer string=w515:string)  [unwired: 1 out]
          n182 = Bundle("Left"=w511, "Top"=w510) -> (w512:cluster{"Left":i32, "Top":i32})  [unwired: 1 out]
          n183 = call "IMAQ Overlay Text"("Text Color (black)"=w514, "error in (no error)"=w520, "String"=w515, "Origin"=w512, "Image"=w518) -> ("error out"=w519:errorcluster, "Image Out"=w523:T9)  [unwired: 3 in, 2 out]
        }
      }
      event "Save Portion of Current Frame": Value Change {
        w531 = FALSE  # Redisplay image
        w532 = FALSE  # Reset control scales?
        n184 = event-data() -> ()  [unwired: 7 out]
        n185 = local read "Acquisition refnum array"() -> (w538:refnum<file>[])
        n186 = local read "Header data"() -> (w536:T2)
        n187 = call "GLIMPSE Save image.vi"("Header data"=w536, "Acqisition files refnums"=w538, "Frame number"=w534) -> ()  [unwired: 2 in, 6 out]
        n188 = local write "Tab Control"(enum32{"Controls", "FOV", "Tools", "Tracking"}."Controls" ("Tab Control")) -> ()
      }
      event "Print Image": Value Change {
        w553 = FALSE  # Redisplay image
        w554 = FALSE  # Reset control scales?
        w567 = "\r"
        # "4- print image"
        n189 = event-data() -> ()  [unwired: 7 out]
        n190 = local write "Tab Control"(enum32{"Controls", "FOV", "Tools", "Tracking"}."Controls" ("Tab Control")) -> ()
        n191 = global read "GLIMPSE Globals.vi" "Current window Black/White Levels"() -> (w570:cluster{ext, ext})
        n192 = property on="Printer" class="Ring (strict)"(error in=w552) -> (error out=w540:errorcluster, "Strings []"=w556:string[])  [unwired: 1 in, 1 out]
        n193 = local read "file path"() -> (w568:path)
        n194 = Unbundle(w570) -> (w561:ext, w562:ext)
        n195 = Number To Decimal String(number=w549) -> (decimal integer string=w559:string)  [unwired: 1 out]
        n196 = Index Array(array=w556, index="Printer") -> (element=w558:string)
        n197 = Path To String(path=w568) -> (string=w569:string)
        n198 = Number To Decimal String(number=w561) -> (decimal integer string=w565:string)  [unwired: 1 out]
        n199 = Number To Decimal String(number=w562) -> (decimal integer string=w563:string)  [unwired: 1 out]
        n200 = Concatenate Strings(w569, w567, "Black: " ("string"), w565, " White: " ("string"), w563, w567, "Frame " ("Printout title"), w559) -> (w543:string)
        n201 = case shown="1, Default" w544 {
          tunnel: w543 -> [w571 w575]
          tunnel: [w571 w576] -> w542
          tunnel: w541 -> [_ w572]
          frame 0 {
          }
          frame 1, Default {
            n202 = Number To Decimal String(number=w572) -> (decimal integer string=w573:string)  [unwired: 1 out]
            n203 = Concatenate Strings(w575, " of FOV " ("string"), w573) -> (w576:string)
          }
        }
        n204 = local read "Overlay?"() -> (w545:bool)
        n205 = call "Print AOI images.vi"("Black/White Levels"=w570, "AOI Overlay?"=w545, "error in (no error)"=w540, "printer name (default)"=w558, "Printout title"=w542, "Image In"=w551) -> ("error out"=w539:errorcluster)  [unwired: 4 out]
      }
      event "Save Sequence": Value Change {
        w586 = FALSE  # Redisplay image
        w587 = FALSE  # Reset control scales?
        n206 = event-data() -> ()  [unwired: 7 out]
        n207 = local read "Acquisition refnum array"() -> (w590:refnum<file>[])
        n208 = global read "GLIMPSE Globals.vi" "Current window Black/White Levels"() -> (w591:cluster{ext, ext})
        n209 = local read "Header data"() -> (w588:T2)
        n210 = local read "Frame Number"() -> (w589:cluster{u32, u32})
        n211 = global write "GLIMPSE Globals.vi" "Sequence range"(w589) -> ()
        n212 = local write "Tab Control"(enum32{"Controls", "FOV", "Tools", "Tracking"}."Controls" ("Tab Control")) -> ()
        n213 = call "GLIMPSE Sequence Save.vi"("Header file data"=w588, "Acquisition refnum array"=w590, "Black/White Levels"=w591) -> ()  [unwired: 1 in, 6 out]
      }
      event "FOV Mode", "Display FOV number", "Total FOVs": Value Change {
        n214 = event-data() -> ()  [unwired: 7 out]
        n215 = property on="Display FOV number" class="Slide (strict)"(error in=w595, "Scale.Maximum"="Total FOVs") -> (error out=w594:errorcluster)  [unwired: 1 in, 1 out]
        n216 = case shown="\"Display one field of view\"" "FOV Mode" {
          tunnel: [w612 i16 1 ("Display FOV number")] -> w605
          tunnel: [w611 i16 0 ("Total FOVs")] -> w606
          tunnel: w598 -> [w615 w616]
          tunnel: [w614 w616] -> w603
          tunnel: "Total FOVs" -> [w611 _]
          tunnel: "Display FOV number" -> [w610 _]
          frame "Display one field of view" {
            n217 = In Range and Coerce(upper limit=w611, x=w610, lower limit=i16 1) -> (coerced(x)=w612:i16)  [unwired: 1 out]
            n218 = Quotient & Remainder(x=w615, y=w611) -> (floor(x/y)=w614:u32)  [unwired: 1 out]
            n219 = local write "Display FOV number"(w612) -> ()
          }
          frame "Display all frames", Default {
          }
        }
        n220 = In Range and Coerce(upper limit=w603, x=w602, lower limit=u32 1) -> (coerced(x)=w599:u32)  [unwired: 1 out]
        n221 = local write "Current Frame Number"(w599) -> ()
      }
      event "Current Frame Number": Value Change {
        w627 = TRUE  # Redisplay image
        w628 = FALSE  # Reset control scales?
        n222 = event-data() -> ()  [unwired: 7 out]
      }
    }
    n223 = case shown="True" w58 {
      tunnel: w39 -> [_ w125]
      tunnel: w49 -> [w121 w127]
      tunnel: [w121 w126] -> w48
      frame False {
      }
      frame True {
        n224 = flat-sequence {
          tunnel: w127 -> [w132]
          tunnel: w125 -> [w128]
          tunnel: [w130] -> w124
          tunnel: [w129] -> w123
          tunnel: [w128] -> w122
          tunnel: [w140] -> w126
          tunnel: w124 -> [w140]
          tunnel: w123 -> [w135]
          tunnel: w122 -> [w134]
          frame #0 {
            w129 = u32 1
            n225 = property on="Current Frame Number" class="Slide (strict)"(error in=w132, "Scale.Range:Maximum"=w128, "Scale.Range:Minimum"=w129, "Maximum"=w128) -> (error out=w131:errorcluster)  [unwired: 1 in, 1 out]
            n226 = property on="Frame Number" class="Slide (strict)"(error in=w131, "Scale.Range:Maximum"=w128, "Scale.Range:Minimum"=w129, "Maximum"=w128) -> (error out=w130:errorcluster)  [unwired: 1 in, 1 out]
          }
          frame #1 {
            n227 = local read "Frame Number"() -> (w139:cluster{u32, u32})
            n228 = Unbundle(w139) -> (w136:u32, w137:u32)
            n229 = In Range and Coerce(upper limit=w134, x=w136, lower limit=w135) -> (coerced(x)=w133:u32)  [unwired: 1 out]
            n230 = Bundle("# of Frames in sequence"=w133, w137) -> (w138:cluster{"# of Frames in sequence":u32, u32})  [unwired: 1 out]
            n231 = local write "Frame Number"(w138) -> ()
          }
        }
      }
    }
    n232 = case shown="True" w50 {
      tunnel: w57 -> [w75 w111]
      tunnel: [errorcluster {"status"=FALSE, "code"=0, "source"=""} ("error out") w104] -> w43
      tunnel: [w75 w100] -> w56
      tunnel: w34 -> [_ w90]
      tunnel: w47 -> [_ w92]
      tunnel: w46 -> [_ w94]
      tunnel: w48 -> [_ w93]
      frame False {
        # "Don't display frame if we are about to quit."
      }
      frame True {
        # "Display frame"
        # "Display current frame"
        n233 = local read "Header2 data"() -> (w89:T1)
        n234 = Decrement(x=w90) -> (x-1=w91:u32)
        n235 = local write "Current Frame Number"(w90) -> ()
        n236 = local read "Header data"() -> (w105:T2)
        n237 = local read "Acquisition refnum array"() -> (w109:refnum<file>[])
        n238 = call "GLIMPSE Fetch Image.vi"("Display FOV number"=w94, "Total FOVs"=w92, "Header file data"=w105, "Acqisition files refnums"=w109, "error in"=w93, "Logical Frame Number\n(starting with zero)"=w91, "Image In"=w111) -> ("error out"=w97:errorcluster, "Image Out"=w99:T9)  [unwired: 2 in, 1 out]
        n239 = Unbundle By Name(w89) -> ("Lasers array"=w88:u16[][], "Filter array"=w86:u16[], "Flow rate array"=w82:dbl[], "Temperature array"=w84:dbl[], "Field array"=w83:u16[])
        n240 = Unbundle By Name(w105) -> ("TTB Array (ms)"=w106:u32[], "Element 0 of TTB"=w107:u32, "Pixel depth"=w102:u32)
        n241 = call "GLIMPSE fetch TTB value.vi"("Array of TTB Values (ms)"=w106, "Logical Frame Number\n(starting with zero)"=w91) -> ("Array index"=w81:u32, "TTB value out"=w108:u32)  [unwired: 5 out]
        "Time\nStamp" <- w108
        n242 = call "Add AOIs overlay to image.vi"("error in (no error)"=w97, "Current frame number\n(starting with 1)"=w90, "Overlay on?"="Overlay?", "Image Src"=w99) -> ("error out"=w96:errorcluster, "Image Dst"=w98:T9)  [unwired: 2 in, 4 out]
        n243 = Index Array(array=w83, index=w81) -> (element=→"Field":u16)
        n244 = Subtract(x=w108, y=w107) -> (x-y=→"Time after 1st\nFrame (ms)":u32)
        n245 = Index Array(array=w84, index=w81) -> (element=→"Temp":dbl)
        n246 = Index Array(array=w86, index=w81) -> (element=→"Filter":u16)
        n247 = Index Array(array=w88, index (row)=w81) -> (element=w87:u16[])  [unwired: 1 in]
        n248 = Index Array(array=w82, index=w81) -> (element=→"Flow":dbl)
        n249 = for {
          N: "# Display\nWindows" -> [_]
          tunnel: w98 -> [w120]
          tunnel: [w119] -> w100
          tunnel: [w118] -> w104
          tunnel: w96 -> [w117]
          tunnel: "Seq. Player" ("Title") -> [w116]
          tunnel: w102 -> [w115]
          i -> [w114]
          n250 = Increment(x=w114) -> (x+1=w113:i32)
          n251 = call "Send image to image display controller.vi"("Image"=w120, "Window Title"=w116, "Window Number"=w113, "error in"=w117, "Image Type"=w115, "Quit display controller?"=FALSE) -> ("Image Out"=w119:T9, "error out"=w118:errorcluster)  [unwired: 1 in, 2 out]
        }
        n252 = Not Equal To 0?(x=w87) -> (x != 0?=→"Lasers":bool[])
      }
    }
    n253 = case shown="\"Play Backward\"" w38 {
      tunnel: [TRUE w72 w73] -> w53
      tunnel: [w69 w72 TRUE] -> w52
      tunnel: [w69 TRUE w73] -> w51
      frame "Stop", Default {
        w69 = FALSE
      }
      frame "Play Forward" {
        w72 = FALSE
      }
      frame "Play Backward" {
        w73 = FALSE
      }
    }
    n254 = Unbundle By Name(w43) -> ("status"=w54:bool)
    n255 = Or(x=w54, y="Exit") -> (x .or. y?=w44:bool)
    n256 = property on="Fwd bkd" class="Bool (strict)"("Visible"=w51) -> ()  [unwired: 2 in, 2 out]
    n257 = property on="Stop bkgd" class="Bool (strict)"("Visible"=w53) -> ()  [unwired: 2 in, 2 out]
    n258 = property on="Rev bkd" class="Bool (strict)"("Visible"=w52) -> ()  [unwired: 2 in, 2 out]
  }
  n259 = stacked-sequence {
    tunnel: w12 -> [w634]
    tunnel: w2 -> [w631]
    tunnel: [w630] -> w1
    frame #0 {
      # "Shutdown"
      n260 = call "IMAQ Dispose"("error in (no error)"=w631) -> ("error out"=w637:errorcluster)  [unwired: 2 in, 3 out]
      n261 = local read "Frame Number"() -> (w635:cluster{u32, u32})
      "Sequence Range" <- w635
      n262 = call "Open caller's caller.vi"("vi reference"=w634) -> ()  [unwired: 1 in, 7 out]
      n263 = call "IMAQ WindToolsClose"("error in (no error)"=w637) -> ("error out"=w632:errorcluster)  [unwired: 5 out]
      n264 = call "Send image to image display controller.vi"("error in"=w632, "Quit display controller?"=TRUE) -> ("error out"=w630:errorcluster)  [unwired: 5 in, 3 out]
      n265 = global write "GLIMPSE Globals.vi" "Sequence range"(w635) -> ()
      n266 = local read "Acquisition refnum array"() -> (w636:refnum<file>[])
      n267 = for {
        tunnel: w636 -> [w638] mode=indexing
        n268 = Close File(refnum=w638) -> ()  [unwired: 1 in, 2 out]
      }
    }
  }
  n269 = call "Glimpse error handler.vi"("error in"=w1) -> ()  [unwired: 1 in, 6 out]
